vi "register panel events.vi"(8 "error in (no error)":errorcluster, 10 "Event Registration Refnum":refnum<event-registration>, 11 "Loop data in":T1 {"PanelMap"."Data"."Plot Bounds (%)"."Bottom (%)" format="%.2f"; "PanelMap"."Data"."Plot Bounds (%)"."Top (%)" format="%.2f"; "PanelMap"."Data"."Plot Bounds (%)"."Right (%)" format="%.2f"; "PanelMap"."Data"."Plot Bounds (%)"."Left (%)" format="%.2f"}) -> (0 "error out":errorcluster, 2 "Event Registration Refnum":refnum<event-registration>, 3 "Loop data out":T1 {"PanelMap"."Data"."Plot Bounds (%)"."Bottom (%)" format="%.2f"; "PanelMap"."Data"."Plot Bounds (%)"."Top (%)" format="%.2f"; "PanelMap"."Data"."Plot Bounds (%)"."Right (%)" format="%.2f"; "PanelMap"."Data"."Plot Bounds (%)"."Left (%)" format="%.2f"})   [LabVIEW 2021, in "MultiRocketPlotPanel.lvclass"]
uses:
  MultiRocketPlotPanel.lvclass
  SubVIs/Loop Data.ctl
  <vilib>/IlluminatedG/IG OOPanel/OOPanel/Manager/Manager.lvclass
  SubVIs/Panel Map.ctl
  SubVIs/Panel Map Data.ctl
  <userlib>/bjustice/RocketPlot/Classes/RocketPlotPanel/RocketPlotPanel.lvclass
  SubVIs/Window Position.ctl
  <vilib>/IlluminatedG/IG OOPanel/OOPanel/Panel/Panel Events.ctl
  <vilib>/IlluminatedG/IG OOPanel/OOPanel/Panel/Visbility Event Data.ctl
  <vilib>/IlluminatedG/IG OOPanel/OOPanel/Visibility State.ctl
  <vilib>/IlluminatedG/IG OOPanel/OOPanel/Close Reason.ctl
  <userlib>/bjustice/RocketPlot/Classes/RocketPlotHandle/SubVIs/callback data.ctl
  <userlib>/bjustice/RocketPlot/Classes/RocketPlotHandle/SubVIs/callback type.ctl
  <userlib>/bjustice/RocketPlot/Classes/RocketPlotPanel/RocketPlotPanel.lvclass/RocketPlotPanel.ctl
  <userlib>/bjustice/RocketPlot/Classes/RocketPlotHandle/RocketPlotHandle.lvclass/RocketPlotHandle.ctl
  <userlib>/bjustice/RocketPlot/Classes/RocketPlotPanel/Read RocketPlotHandle.vi
  <userlib>/bjustice/RocketPlot/Classes/RocketPlotHandle/Read callback UE.vi
  <userlib>/bjustice/RocketPlot/Classes/RocketPlotHandle/RocketPlotHandle.lvclass
  <vilib>/IlluminatedG/IG OOPanel/OOPanel/OOPanel.lvlib
  <vilib>/IlluminatedG/IG OOPanel/OOPanel/Panel/Panel.lvclass
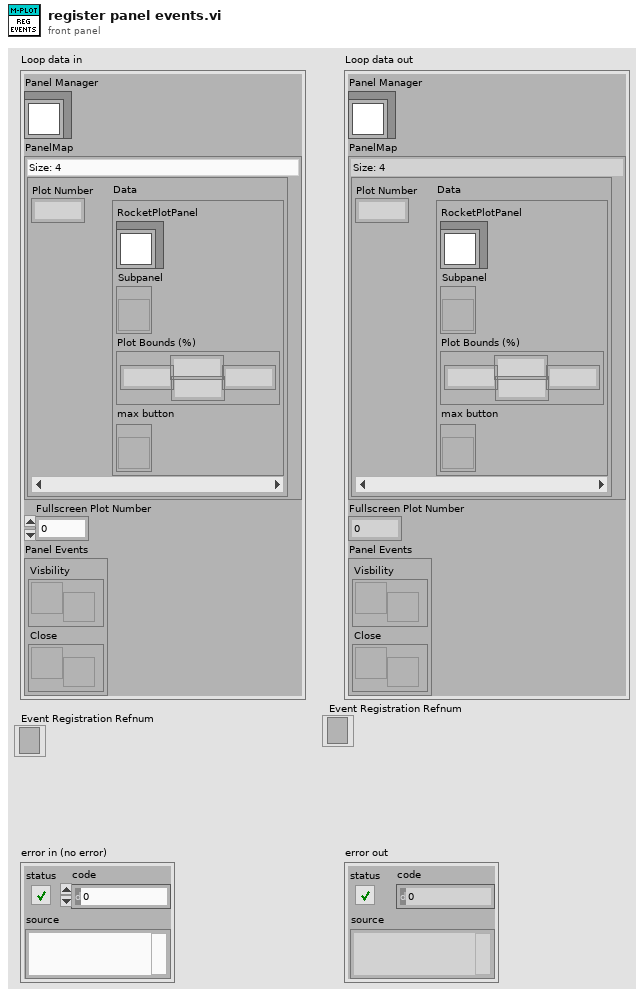
[diagram p1: front panel]
types:
  T1 = typedef "MultiRocketPlotPanel.lvclass/Loop Data.ctl" = cluster{"Panel Manager":refnum<class "Manager.lvclass">, "PanelMap":T2, "Fullscreen Plot Number":i32, "Panel Events":T5}
  T2 = typedef "MultiRocketPlotPanel.lvclass/Panel Map.ctl" = map{i32, T3}
  T3 = typedef "MultiRocketPlotPanel.lvclass/Panel Map Data.ctl" = cluster{"RocketPlotPanel":refnum<class "RocketPlotPanel.lvclass">, "Subpanel":refnum<vi>, "Plot Bounds (%)":T4, "max button":refnum<vi>}
  T4 = typedef "MultiRocketPlotPanel.lvclass/Window Position.ctl" = cluster{"Left (%)":dbl, "Top (%)":dbl, "Right (%)":dbl, "Bottom (%)":dbl}
  T5 = typedef "OOPanel.lvlib/Panel.lvclass/Panel Events.ctl" = cluster{"Visbility":refnum<user-event>, "Close":refnum<user-event>}
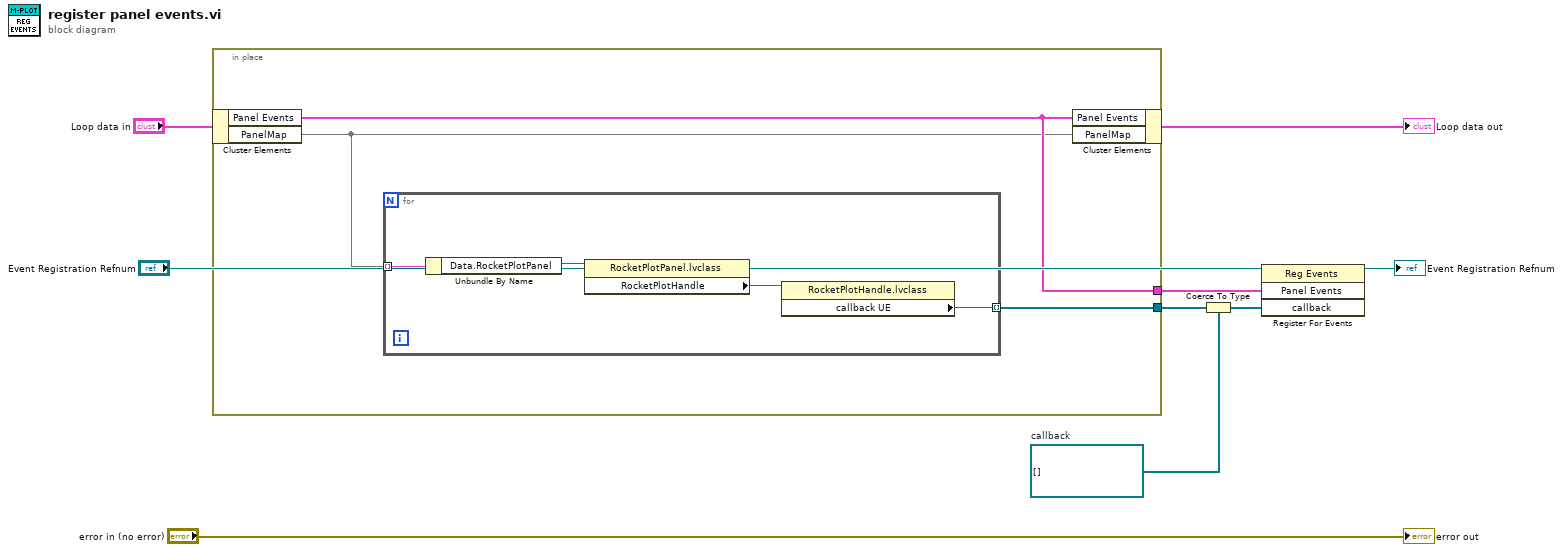
[diagram p0: block diagram]
diagram:
  w4 = refnum<user-event>[] []  # callback
  n1 = in-place {
    in-place-border: [w12] -> w7
    in-place-border: [w10] -> w5
    n2 = in-place-cluster #1("Loop data in") -> ("Panel Events"=w12:T5, "PanelMap"=w11:T2)
    n3 = for {
      tunnel: w11 -> [w16] mode=indexing
      tunnel: [w13] -> w10 mode=indexing
      n4 = Unbundle By Name(w16) -> ("Data.RocketPlotPanel"=w15:refnum<class "RocketPlotPanel.lvclass">)
      n5 = property class="RocketPlotPanel.lvclass"(reference=w15) -> ("RocketPlotHandle"=w14:refnum<class "RocketPlotHandle.lvclass">)  [unwired: 1 in, 2 out]
      n6 = property class="RocketPlotHandle.lvclass"(reference=w14) -> ("callback UE"=w13:refnum<user-event>)  [unwired: 1 in, 2 out]
    }
    n7 = in-place-cluster #1("Panel Events"=w12, "PanelMap"=w11) -> (→"Loop data out":T1)
  }
  n8 = Coerce To Type(0:w5, 1:w4) -> (2:w3:refnum<user-event>[])
  n9 = register-events(reference="Event Registration Refnum", w7, w3) -> (reference out=→"Event Registration Refnum":refnum<event-registration>)  [unwired: 1 in, 1 out]
  "error out" <- "error in (no error)"
